vi "Test.Runner.vi"() -> ()   [LabVIEW 2025]
uses:
  submodules/Market.Data.Common/fpga/orderbook.command.ctl
  submodules/Market.Data.Common/fpga/orderbook.command.type.ctl
  <vilib>/rvi/interface/RandomDataEmulation/nirviRandomDataOpen.vi
  <vilib>/rvi/interface/common/niFpgaCacheSessionInfoDynamic.vi
  <vilib>/FPGAPlugInAG/Dynamic/niLvFpga_Run_Dynamic.vi
  <vilib>/Utility/error.llb/Error Cluster From Error Code.vi
  <vilib>/rvi/errors/niLvFpgaAdjustHostInterfaceError.vi
  <vilib>/FPGAPlugInAG/Dynamic/niLvFpga_Close_Dynamic.vi
  <vilib>/rvi/interface/nirviOpenFPGA/nirviOpenFPGA.xnode
  fpga/poc.ip.vi
  <vilib>/rvi/interface/nirviMethod/nirviMethod.xnode
  <vilib>/rvi/interface/nirviReadWriteControl/nirviReadWriteControl.xnode
  <vilib>/rvi/interface/nirviCloseFPGA/nirviCloseFPGA.xnode
  <vilib>/rvi/errors/niLvFpgaMergeErrorWithErrorCode.vi
  <vilib>/FPGAPlugInAG/Dynamic/niLvFpga_ReadFifo_Dynamic.vi
  <vilib>/rvi/interface/Simulation/niFpgaSimulationCallBeginRW.vi
  submodules/Market.Data.Common/host/fpganow.common.host.lvlib
  NiFpgaLv.dll
  <vilib>/FPGAPlugInAG/Dynamic/niLvFpga_WriteFifo_Dynamic.vi
  submodules/Market.Data.Common/fpga/fpganow.common.fpga.lvlib
panel:
  out "MDebug":u64[][](array[numeric]) format="%.0x"
  out "Ob.cmd [str]":string[](array[string])
  out "Data Sent 3":u64[][](array[numeric]) format="%016x"
  out "Debug":u64[][](array[numeric]) format="%.0x"
  out "Deserialized\nOrderBook.Commands":u64[](array[numeric]) format="%.0x"
  out "OrderBook.Command[]":T1[](array[typedef]) {"price" format="%.0x"; "symbol" format="%.0x"; "orderId" format="%.0x"; "side" format="%.0x"}
  out "error out":errorcluster
  in  "error in":errorcluster
  in  "Raw_Data File Path":path=path "C:/work/fpganow/Market.Data.PoC/submodules/cboe_pitch/generated_2025_05_06.pcap"
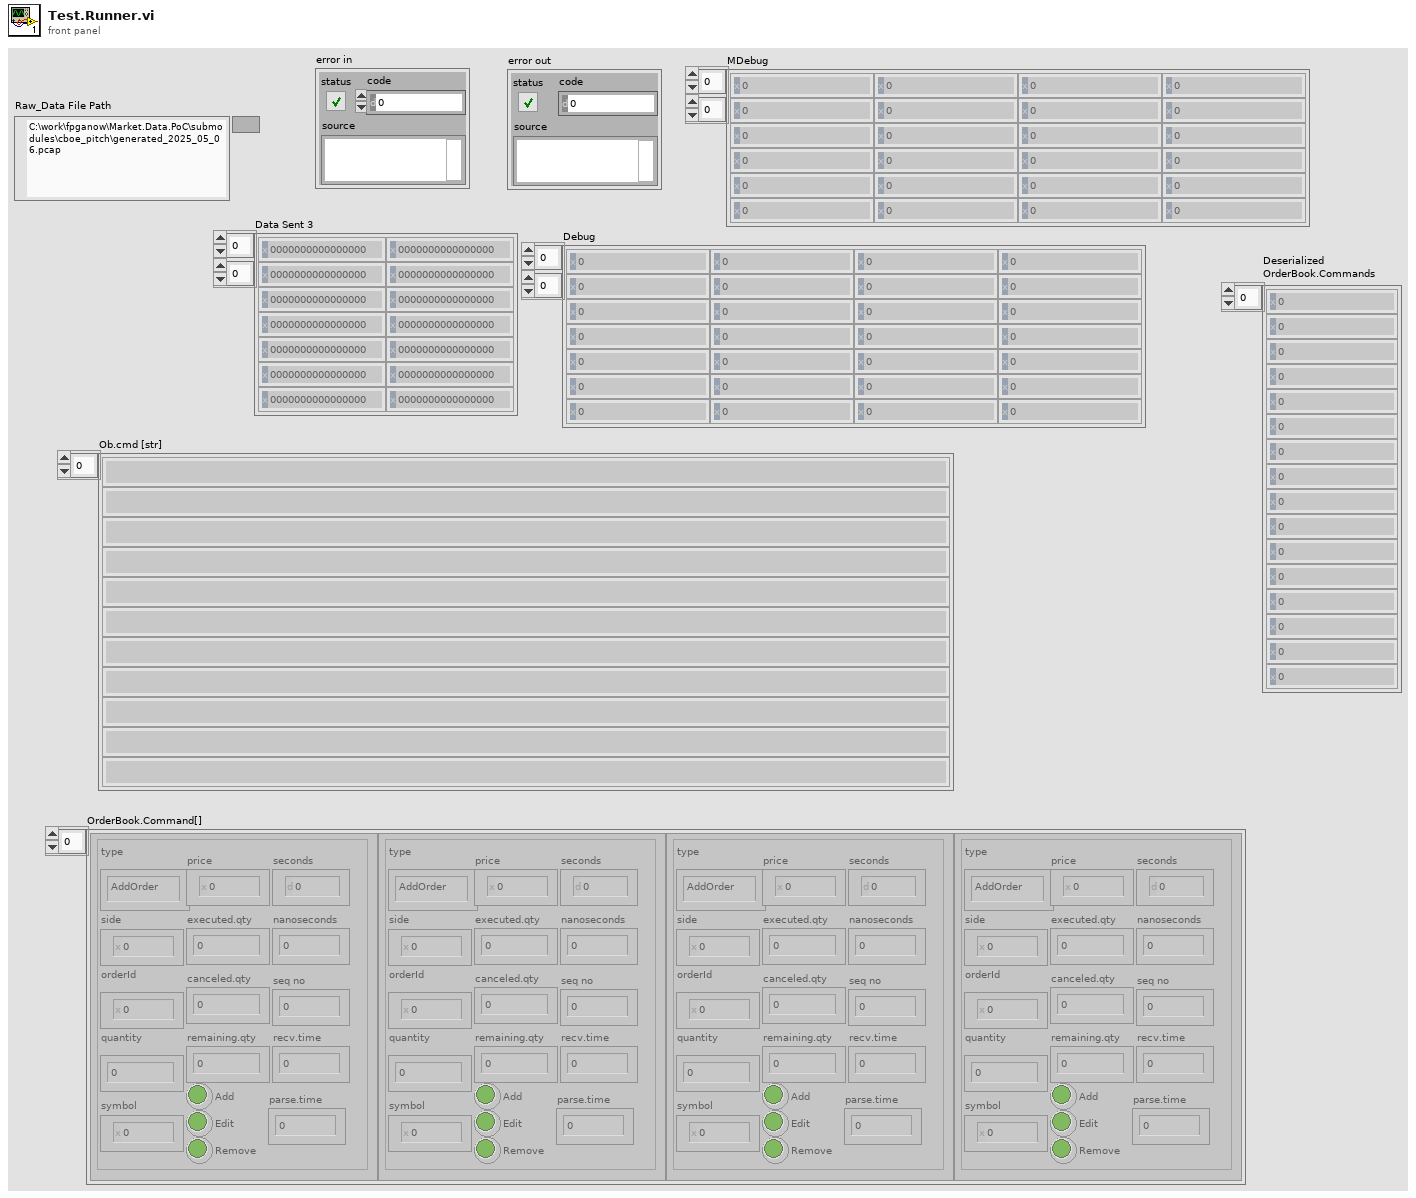
[diagram p1: front panel]
types:
  T1 = typedef "fpganow.common.fpga.lvlib/orderbook.command.ctl" = cluster{"type":T2, "side":u8, "orderId ":u64, "quantity":u32, "symbol":u64, "price":u64, "executed.qty":u32, "canceled.qty":u32, "remaining.qty":u32, "seconds":u64, "nanoseconds":u64, "Add":bool, "Edit":bool, "Remove":bool, "seq no":u32, "recv.time":u64, "parse.time":u64}
  T2 = typedef "fpganow.common.fpga.lvlib/orderbook.command.type.ctl" = enum8{"Time", "AddOrder", "OrderExecuted", "OrderExecutedAtPrice", "ReduceSize", "ModifyOrder", "DeleteOrder", "Get.Everything", "Get.All.Orders", "Get.Top"}
  T3 = typedef "record.ctl" = cluster{"ts_sec":u32, "ts_usec":u32, "incl_len":u32, "orig_len":u32, "payload":u8[]}
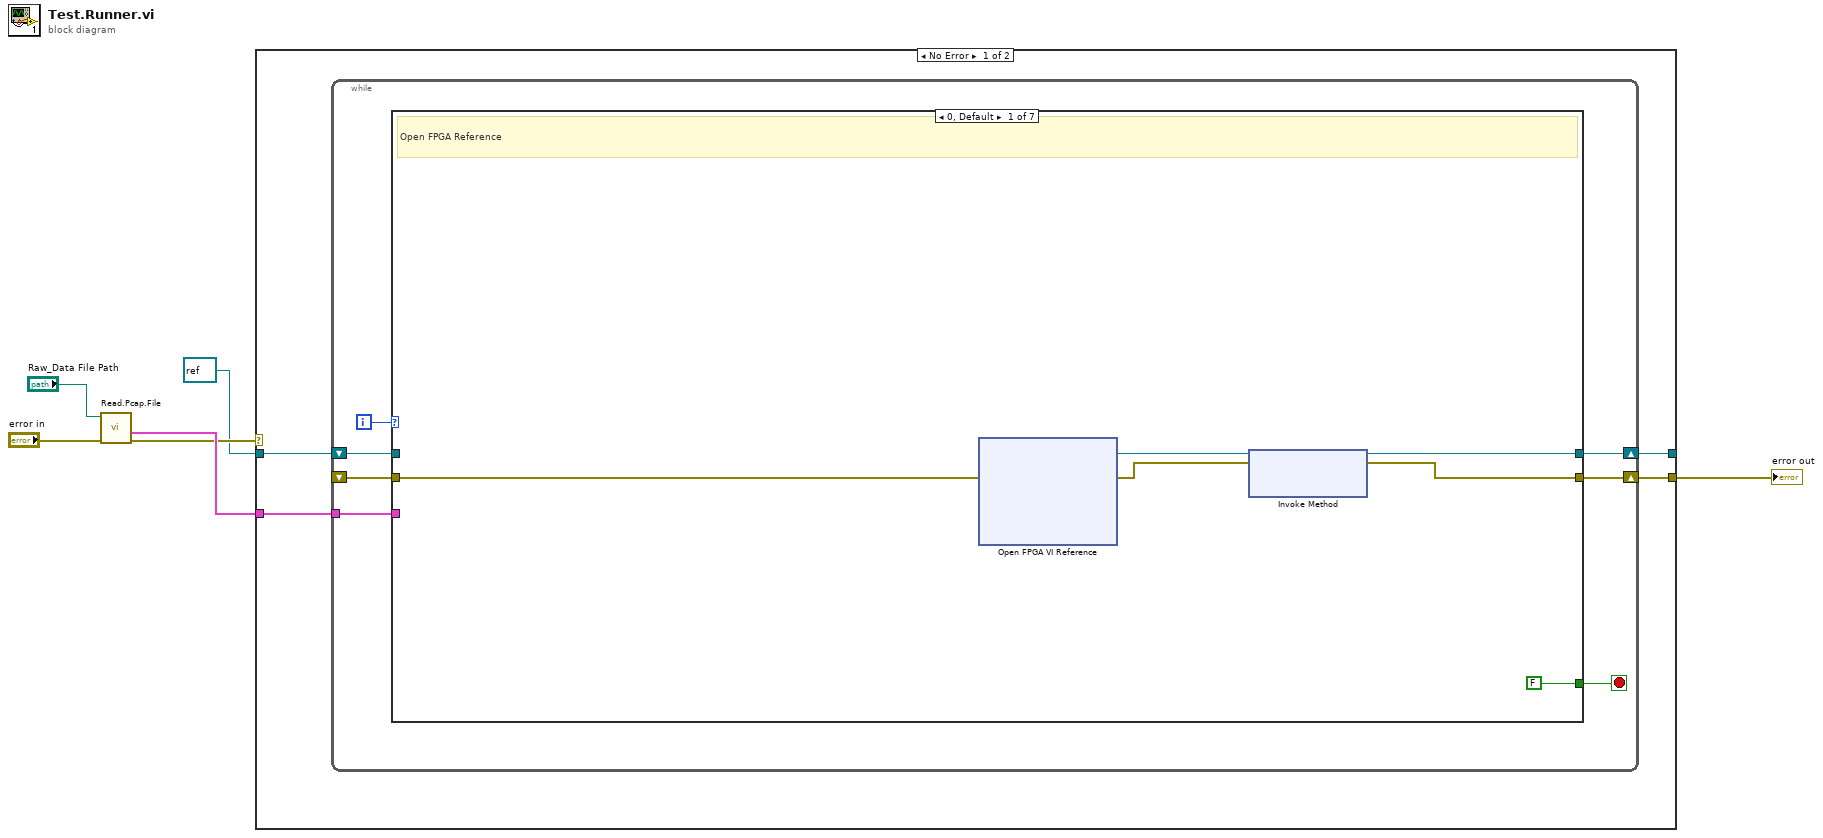
[diagram p0: block diagram]
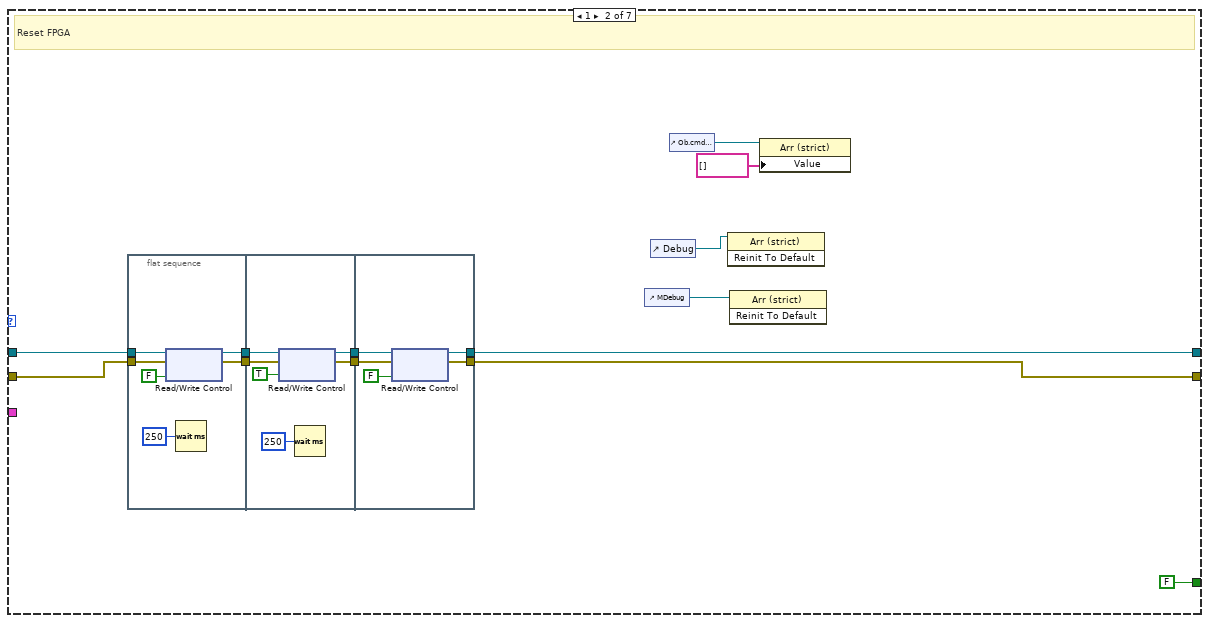
[diagram p2: hidden frame]
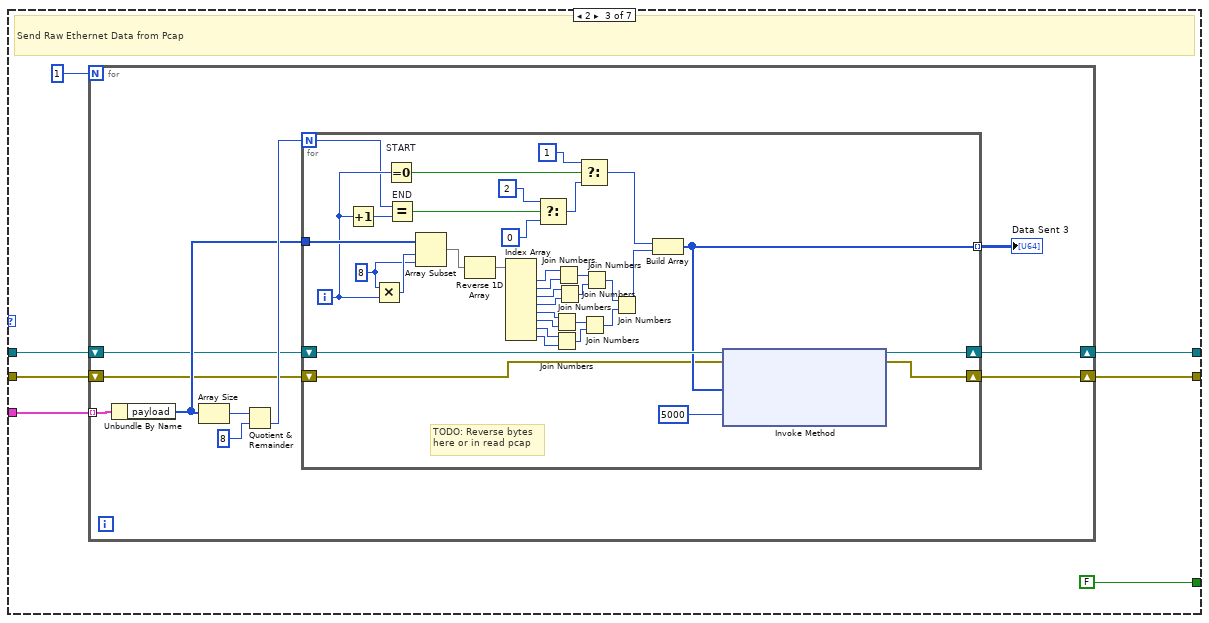
[diagram p3: hidden frame]
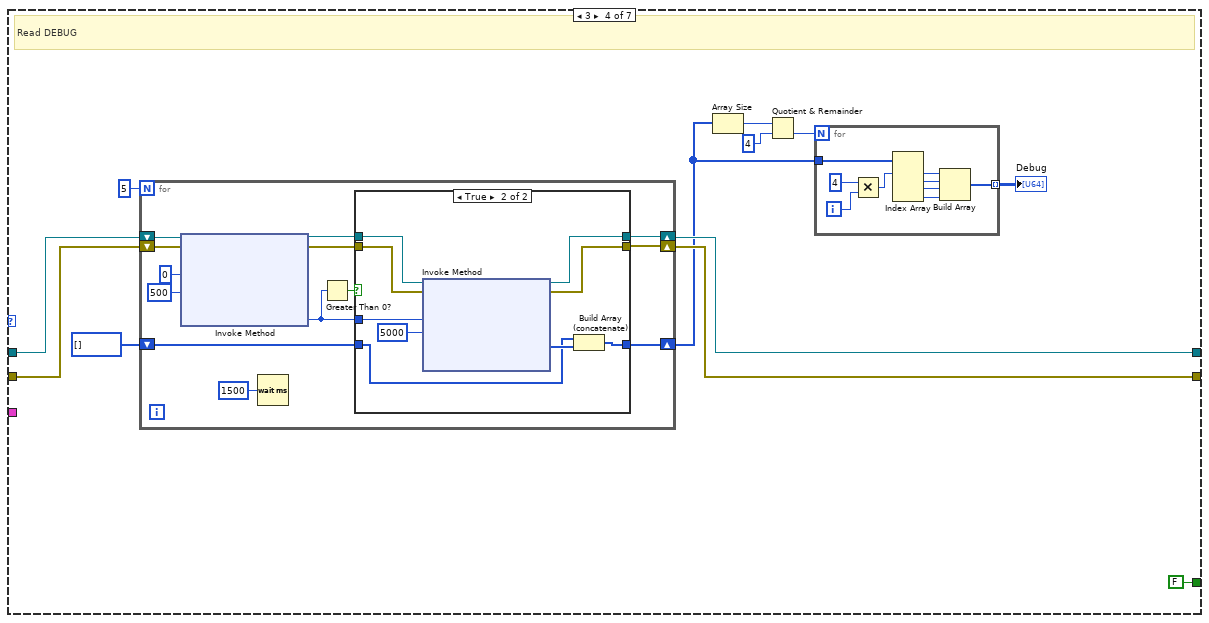
[diagram p4: hidden frame]
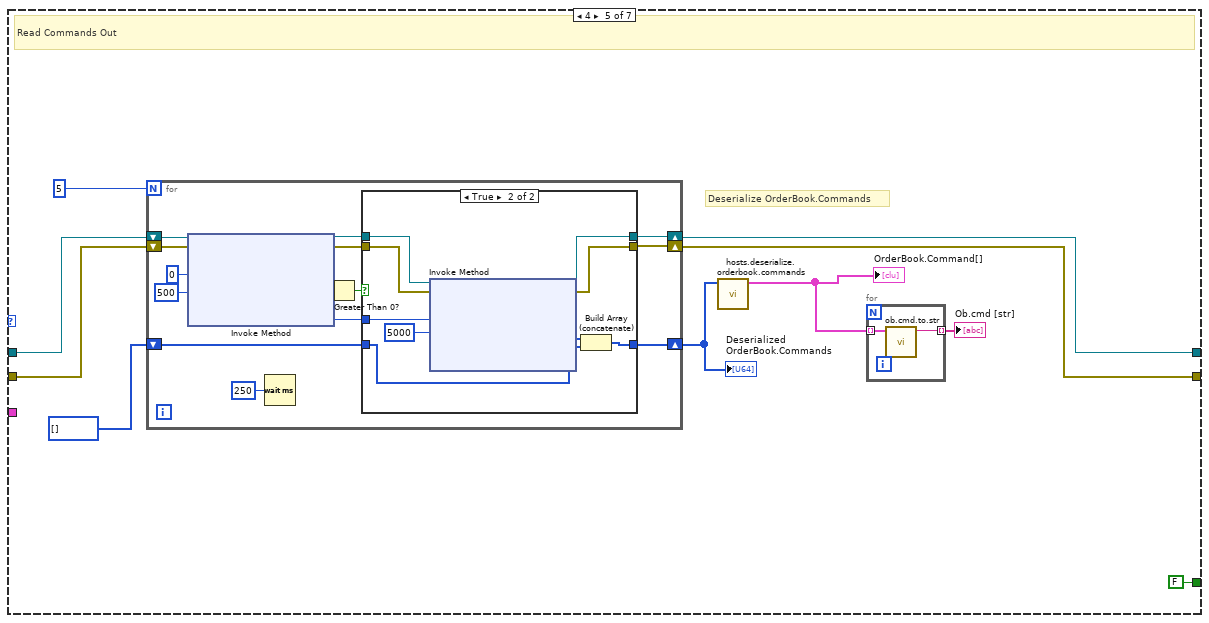
[diagram p6: hidden frame]
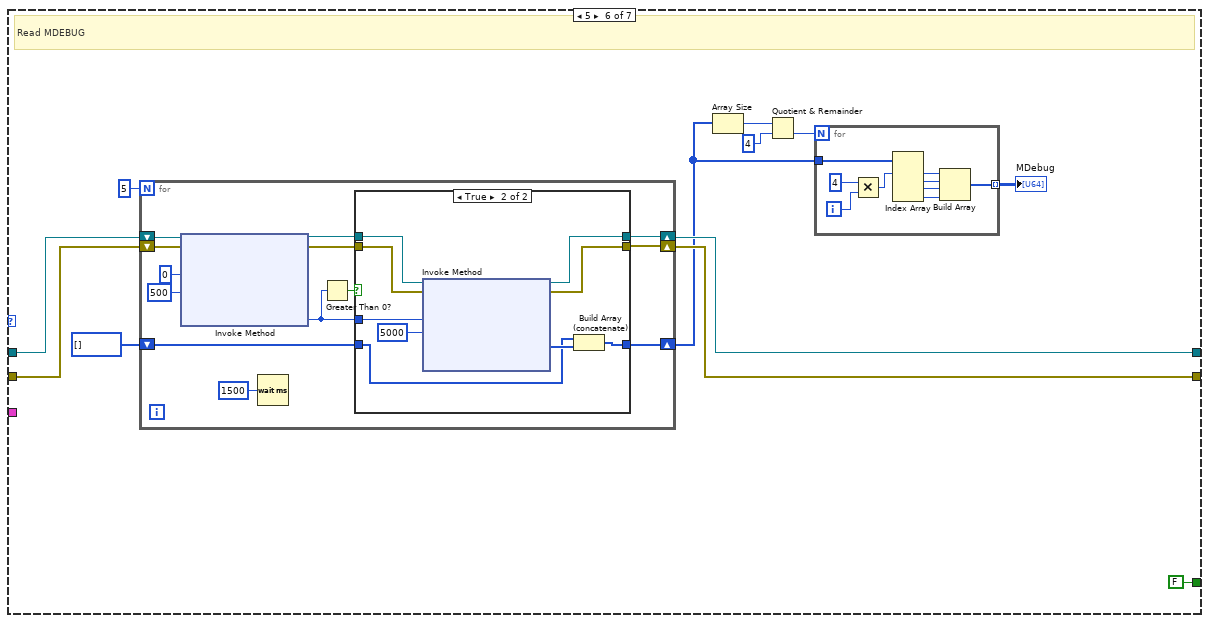
[diagram p8: hidden frame]
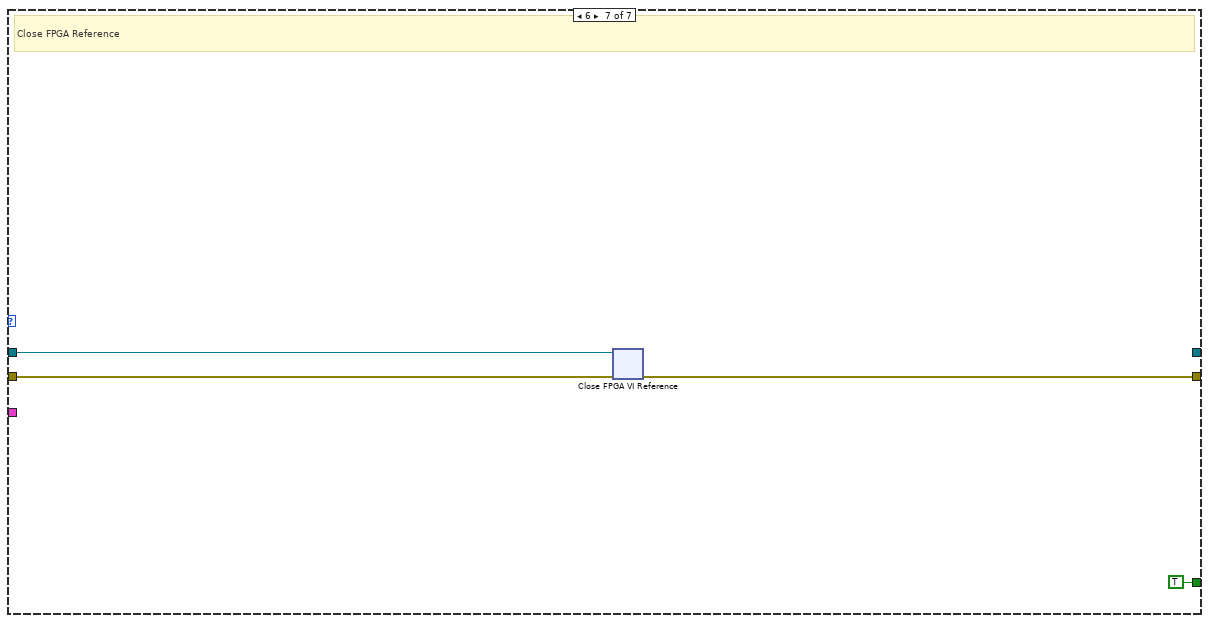
[diagram p10: hidden frame]
diagram:
  n1 = call "Read.Pcap.File.vi"("error in"="error in", "Path"="Raw_Data File Path") -> ("error out"=w4:errorcluster, "Records"=w5:T3[])  [unwired: 6 in, 2 out]
  n2 = case shown="No Error" w4 {
    selector: w4 -> [_ w240]
    tunnel: w5 -> [w10 _]
    tunnel: refnum<k20> refnum ("FPGA VI Reference Out") -> [w9 _]
    tunnel: [w8 _] -> _
    tunnel: [w7 w240] -> w3
    frame No Error {
      n3 = while {
        tunnel: w10 -> [w17]
        shift-right: [w11] -> w8
        shift-left: w9 -> [w16]
        shift-right: [w15] -> w7
        shift-left: _ -> [w14]
        i -> [w13]
        stop <- w12 stop-if-true
        n4 = case shown="0, Default" w13 {
          tunnel: w17 -> [_ _ w55 _ _ _ _]
          tunnel: w16 -> [_ w36 w60 w118 w161 w201 w239]
          tunnel: [w19 w35 w59 w115 w158 w198 _] -> w11
          tunnel: [w18 w34 w58 w114 w157 w197 w237] -> w15
          tunnel: w14 -> [w22 w33 w57 w116 w159 w199 w238]
          tunnel: [FALSE FALSE FALSE FALSE FALSE FALSE TRUE] -> w12
          frame 0, Default {
            # "Open FPGA Reference"
            n5 = xnode "Open FPGA VI Reference"("error in"=w22) -> ("FPGA VI Reference Out"=w21:refnum<k20>, "error out"=w20:errorcluster)  [unwired: 1 in]
            n6 = xnode "Invoke Method"("FPGA VI Reference In"=w21, "error in"=w20) -> ("FPGA VI Reference Out"=w19:refnum<k20>, "error out"=w18:errorcluster)  [unwired: 1 in]
          }
          frame 1 {
            # "Reset FPGA"
            n7 = flat-sequence {
              tunnel: w36 -> [w42]
              tunnel: w33 -> [w39]
              tunnel: [w41] -> w31
              tunnel: [w40] -> w30
              tunnel: w31 -> [w47]
              tunnel: w30 -> [w48]
              tunnel: [w45] -> w29
              tunnel: [w46] -> w28
              tunnel: [w51] -> w34
              tunnel: [w50] -> w35
              tunnel: w29 -> [w52]
              tunnel: w28 -> [w53]
              frame #0 {
                n8 = xnode "Read/Write Control"("FPGA VI Reference In"=w42, "error in"=w39, "ip.reset"=FALSE ("Reset")) -> ("FPGA VI Reference Out"=w41:refnum<k20>, "error out"=w40:errorcluster)
                n9 = Wait (ms)(milliseconds to wait=u32 250) -> ()  [unwired: 1 out]
              }
              frame #1 {
                n10 = xnode "Read/Write Control"("FPGA VI Reference In"=w47, "error in"=w48, "ip.reset"=TRUE ("Reset")) -> ("FPGA VI Reference Out"=w45:refnum<k20>, "error out"=w46:errorcluster)
                n11 = Wait (ms)(milliseconds to wait=u32 250) -> ()  [unwired: 1 out]
              }
              frame #2 {
                n12 = xnode "Read/Write Control"("FPGA VI Reference In"=w52, "error in"=w53, "ip.reset"=FALSE ("Reset")) -> ("FPGA VI Reference Out"=w50:refnum<k20>, "error out"=w51:errorcluster)
              }
            }
            n13 = control-ref of="MDebug"() -> (w27:refnum<vi>)
            n14 = control-ref of="Debug"() -> (w26:refnum<vi>)
            n15 = control-ref of="Ob.cmd [str]"() -> (w25:refnum<vi>)
            n16 = invoke class="Arr (strict)" method="Reinit To Default"(reference=w26) -> ()  [unwired: 2 in, 3 out]
            n17 = invoke class="Arr (strict)" method="Reinit To Default"(reference=w27) -> ()  [unwired: 2 in, 3 out]
            n18 = property class="Arr (strict)"(reference=w25, "Value"=string[] []) -> ()  [unwired: 1 in, 2 out]
          }
          frame 2 {
            # "Send Raw Ethernet Data from Pcap"
            n19 = for {
              N: 1 -> [_]
              tunnel: w55 -> [w66] mode=indexing
              shift-right: [w64] -> w59
              shift-left: w60 -> [w63]
              shift-right: [w62] -> w58
              shift-left: w57 -> [w61]
              n20 = Unbundle By Name(w66) -> ("payload"=w67:u8[])
              n21 = Array Size(array=w67) -> (size(s)=w70:i32)
              n22 = Quotient & Remainder(x=w70, y=8) -> (floor(x/y)=w68:i32)  [unwired: 1 out]
              n23 = for {
                N: w68 -> [w102]
                tunnel: w67 -> [w104]
                tunnel: [w76] -> w65 mode=indexing
                shift-right: [w78] -> w64
                shift-left: w63 -> [w77]
                shift-right: [w74] -> w62
                shift-left: w61 -> [w73]
                i -> [w103]
                w105 = 8 ("x")
                # "TODO: Reverse bytes\nhere or in read pcap"
                n24 = Increment(x=w103) -> (x+1=w101:i32)
                n25 = Multiply(x=w105, y=w103) -> (x*y=w106:i32)
                n26 = Equal To 0? "START"(x=w103) -> (x = 0?=w100:bool)
                n27 = Equal? "END"(x=w102, y=w101) -> (x = y?=w98:bool)
                n28 = Array Subset(array=w104, index=w106, length=w105) -> (w71:u8[])
                n29 = Reverse 1D Array(array=w71) -> (reversed array=w72:u8[])
                n30 = Index Array(array=w72) -> (element #1=w93:u8, element #2=w94:u8, element #3=w92:u8, element #4=w91:u8, element #5=w89:u8, element #6=w90:u8, element #7=w88:u8, element #8=w87:u8)  [unwired: 8 in]
                n31 = Select(t=u64 2, s=w98, f=u64 0) -> (s? t:f=w95:u64)
                n32 = Join Numbers(hi=w89, lo=w90) -> ((hi.lo)=w84:u16)
                n33 = Join Numbers(hi=w88, lo=w87) -> ((hi.lo)=w83:u16)
                n34 = Join Numbers(hi=w93, lo=w94) -> ((hi.lo)=w86:u16)
                n35 = Join Numbers(hi=w92, lo=w91) -> ((hi.lo)=w85:u16)
                n36 = Select(t=u64 1, s=w100, f=w95) -> (s? t:f=w79:u64)
                n37 = Join Numbers(hi=w84, lo=w83) -> ((hi.lo)=w81:u32)
                n38 = Join Numbers(hi=w86, lo=w85) -> ((hi.lo)=w82:u32)
                n39 = Join Numbers(hi=w82, lo=w81) -> ((hi.lo)=w80:u64)
                n40 = Build Array(w79, w80) -> (w76:u64[])
                n41 = xnode "Invoke Method"("FPGA VI Reference In"=w77, "error in"=w73, "Data"=w76, "Timeout (ms)"=5000) -> ("FPGA VI Reference Out"=w78:refnum<k20>, "error out"=w74:errorcluster)  [unwired: 1 out]
              }
              "Data Sent 3" <- w65
            }
          }
          frame 3 {
            # "Read DEBUG"
            n42 = for {
              N: 5 -> [_]
              shift-right: [w134] -> w115
              shift-left: w118 -> [w140]
              shift-right: [w133] -> w114
              shift-left: w116 -> [w139]
              shift-right: [w135] -> w110
              shift-left: u64[] [] -> [w129]
              n43 = xnode "Invoke Method"("FPGA VI Reference In"=w140, "error in"=w139, "Number of Elements"=u32 0, "Timeout (ms)"=500) -> ("FPGA VI Reference Out"=w132:refnum<k20>, "error out"=w131:errorcluster, "Elements Remaining"=w130:u32)  [unwired: 1 out]
              n44 = Wait (ms)(milliseconds to wait=u32 1500) -> ()  [unwired: 1 out]
              n45 = Greater Than 0?(x=w130) -> (x > 0?=w136:bool)
              n46 = case shown="True" w136 {
                tunnel: [w141 w151] -> w135
                tunnel: [w143 w150] -> w134
                tunnel: [w142 w149] -> w133
                tunnel: w132 -> [w143 w148]
                tunnel: w131 -> [w142 w147]
                tunnel: w130 -> [_ w146]
                tunnel: w129 -> [w141 w144]
                frame False {
                }
                frame True {
                  n47 = xnode "Invoke Method"("FPGA VI Reference In"=w148, "error in"=w147, "Number of Elements"=w146, "Timeout (ms)"=5000) -> ("FPGA VI Reference Out"=w150:refnum<k20>, "error out"=w149:errorcluster, "Data"=w152:u64[])  [unwired: 1 out]
                  n48 = Build Array (concatenate)(w144, w152) -> (w151:u64[])
                }
              }
            }
            n49 = Array Size(array=w110) -> (size(s)=w112:i32)
            n50 = Quotient & Remainder(x=w112, y=4) -> (floor(x/y)=w108:i32)  [unwired: 1 out]
            n51 = for {
              N: w108 -> [_]
              tunnel: w110 -> [w127]
              tunnel: [w119] -> w109 mode=indexing
              i -> [w126]
              n52 = Multiply(x=4, y=w126) -> (x*y=w125:i32)
              n53 = Index Array(array=w127, index #1=w125) -> (element #1=w123:u64, element #2=w120:u64, element #3=w121:u64, element #4=w122:u64)  [unwired: 3 in]
              n54 = Build Array(w123, w120, w121, w122) -> (w119:u64[])
            }
            "Debug" <- w109
          }
          frame 4 {
            # "Deserialize OrderBook.Commands"
            # "Read Commands Out"
            n55 = for {
              N: 5 -> [_]
              shift-right: [w171] -> w158
              shift-left: w161 -> [w177]
              shift-right: [w170] -> w157
              shift-left: w159 -> [w176]
              shift-right: [w172] -> w155
              shift-left: u64[] [] -> [w166]
              n56 = xnode "Invoke Method"("FPGA VI Reference In"=w177, "error in"=w176, "Number of Elements"=u32 0, "Timeout (ms)"=500) -> ("FPGA VI Reference Out"=w169:refnum<k20>, "error out"=w168:errorcluster, "Elements Remaining"=w167:u32)  [unwired: 1 out]
              n57 = Wait (ms)(milliseconds to wait=u32 250) -> ()  [unwired: 1 out]
              n58 = Greater Than 0?(x=w167) -> (x > 0?=w173:bool)
              n59 = case shown="True" w173 {
                tunnel: [w178 w188] -> w172
                tunnel: [w180 w187] -> w171
                tunnel: [w179 w186] -> w170
                tunnel: w169 -> [w180 w185]
                tunnel: w168 -> [w179 w184]
                tunnel: w167 -> [_ w183]
                tunnel: w166 -> [w178 w181]
                frame False {
                }
                frame True {
                  n60 = xnode "Invoke Method"("FPGA VI Reference In"=w185, "error in"=w184, "Number of Elements"=w183, "Timeout (ms)"=5000) -> ("FPGA VI Reference Out"=w187:refnum<k20>, "error out"=w186:errorcluster, "Data"=w189:u64[])  [unwired: 1 out]
                  n61 = Build Array (concatenate)(w181, w189) -> (w188:u64[])
                }
              }
            }
            "Deserialized\nOrderBook.Commands" <- w155
            n62 = call "hosts.deserialize.orderbook.commands.vi"("DataIn"=w155) -> ("OrderBook.Command[]"=w153:T1[])  [unwired: 10 in]
            "OrderBook.Command[]" <- w153
            n63 = for {
              tunnel: w153 -> [w164] mode=indexing
              tunnel: [w163] -> w154 mode=indexing
              n64 = call "ob.cmd.to.str.vi"("orderbook.command"=w164) -> ("string"=w163:string)  [unwired: 10 in]
            }
            "Ob.cmd [str]" <- w154
          }
          frame 5 {
            # "Read MDEBUG"
            n65 = for {
              N: 5 -> [_]
              shift-right: [w217] -> w198
              shift-left: w201 -> [w223]
              shift-right: [w216] -> w197
              shift-left: w199 -> [w222]
              shift-right: [w218] -> w193
              shift-left: u64[] [] -> [w212]
              n66 = xnode "Invoke Method"("FPGA VI Reference In"=w223, "error in"=w222, "Number of Elements"=u32 0, "Timeout (ms)"=500) -> ("FPGA VI Reference Out"=w215:refnum<k20>, "error out"=w214:errorcluster, "Elements Remaining"=w213:u32)  [unwired: 1 out]
              n67 = Wait (ms)(milliseconds to wait=u32 1500) -> ()  [unwired: 1 out]
              n68 = Greater Than 0?(x=w213) -> (x > 0?=w219:bool)
              n69 = case shown="True" w219 {
                tunnel: [w224 w234] -> w218
                tunnel: [w226 w233] -> w217
                tunnel: [w225 w232] -> w216
                tunnel: w215 -> [w226 w231]
                tunnel: w214 -> [w225 w230]
                tunnel: w213 -> [_ w229]
                tunnel: w212 -> [w224 w227]
                frame False {
                }
                frame True {
                  n70 = xnode "Invoke Method"("FPGA VI Reference In"=w231, "error in"=w230, "Number of Elements"=w229, "Timeout (ms)"=5000) -> ("FPGA VI Reference Out"=w233:refnum<k20>, "error out"=w232:errorcluster, "Data"=w235:u64[])  [unwired: 1 out]
                  n71 = Build Array (concatenate)(w227, w235) -> (w234:u64[])
                }
              }
            }
            n72 = Array Size(array=w193) -> (size(s)=w195:i32)
            n73 = Quotient & Remainder(x=w195, y=4) -> (floor(x/y)=w191:i32)  [unwired: 1 out]
            n74 = for {
              N: w191 -> [_]
              tunnel: w193 -> [w210]
              tunnel: [w202] -> w192 mode=indexing
              i -> [w209]
              n75 = Multiply(x=4, y=w209) -> (x*y=w208:i32)
              n76 = Index Array(array=w210, index #1=w208) -> (element #1=w206:u64, element #2=w203:u64, element #3=w204:u64, element #4=w205:u64)  [unwired: 3 in]
              n77 = Build Array(w206, w203, w204, w205) -> (w202:u64[])
            }
            "MDebug" <- w192
          }
          frame 6 {
            # "Close FPGA Reference"
            n78 = xnode "Close FPGA VI Reference"("FPGA VI Reference In"=w239, "error in"=w238) -> ("error out"=w237:errorcluster)
          }
        }
      }
    }
    frame Error {
    }
  }
  "error out" <- w3
